vi "HMI.vi"() -> ()   [LabVIEW 2019, in "HMI Class 3.lvclass"]
uses:
  HMI Class 3.lvclass
  Control2.ctl
  Class 2.lvclass
  Datos Out.vi
  Datos In.vi
panel:
  out "mensajes a usuario":string
  in  "PARO DE E":bool
  in  "HISTORIAL DE FALLAS":bool
  in  "MODO AUTOMATICO":T1
  in  "Test":bool
  out "Numeric":dbl
  in  "MODO MANUAL":bool
  in  "stop":bool
  in  "INICIO":bool
  out "FALLA PRESENTE":bool
  out "MAQUINA EN ORIGEN":bool
  in  "RESET":bool
  in  "Tab Control":enum32{"0", "1", "2", "3", "4", "6", "7"}(tab)
  in  "MOVER A ORIGEN":bool
  out "PIEZA 2":bool
  out "PIEZA":bool
  in  "LIMITE MINIMO 2":dbl min=0.0 max=9999.0
  in  "LIMITE MAXIMO 2":dbl min=0.0 max=9999.0
  in  "LIMITE MINIMO":dbl min=0.0 max=9999.0
  in  "LIMITE MAXIMO":dbl min=0.0 max=9999.0
  out "ESTADO DE PIEZA TENSION":string
  out "ESTADO DE PIEZA GAP":string
  out "VALOR DE DISTANCIA":dbl
  in  "EST 2":bool
  out "SIN CAMBIOS":bool
  out "CON CAMBIOS":bool
  in  "EST 3":bool
  out "VALOR DE TENSIÓN":dbl
  in  "EST 1":bool
  out "SMAC SEGURO":bool
  out "PIEZA EN NIDO":bool
  in  "MANUAL":bool
  out "SMAC MUESTRA":bool
  out "SMAC APROX":bool
  in  "SMAC AVANZANDO":bool
  in  "SMAC RETORNANDO":bool
  in  "CILINDRO 2":bool
  in  "CILINDRO 1":bool
  out "SMAC AV. SEGURO":bool
  out "SMAC HOME":bool
  out "BIMANUAL 2":bool
  out "BIMANUAL 1":bool
  out "AVANCE CILINDRO 2":bool
  out "HOME CILINDRO 2":bool
  out "AVANCE CILINDRO 1":bool
  out "HOME CILINDRO 1":bool
  in  "ESTADISTICAS DE PRODUCCION":bool
  in  "CONFIGRUARCION DE PARAMETROS":bool
  in  "MODO DE OPERACION 2":bool
  # "MENÚ PRINCIPAL"
  # "MODO DE OPERACIÓN"
  # "ESTACION 1\n PRUEBA TENSIÓN"
  # "ESTACION 2\n PRUEBA GAP"
  # "ESTACION 3\n PRUEBA TRIP-GAP"
  # "CONTINUAIDAD EN CONTACTOS"
  # "PRODUCCIÓN"
  # "SENSORES"
  # "CILINDROS"
  # "SEGURIDAD"
  # "ESTADO DEL SMAC"
  # "SMAC"
  # "ENTRADAS                        SALIDAS"
  # "CONFIGURACION DE PARAMETROS"
  # "ESTADISTICAS DE PRODUCCIÓN"
  # "HISTORIAL DE FALLAS"
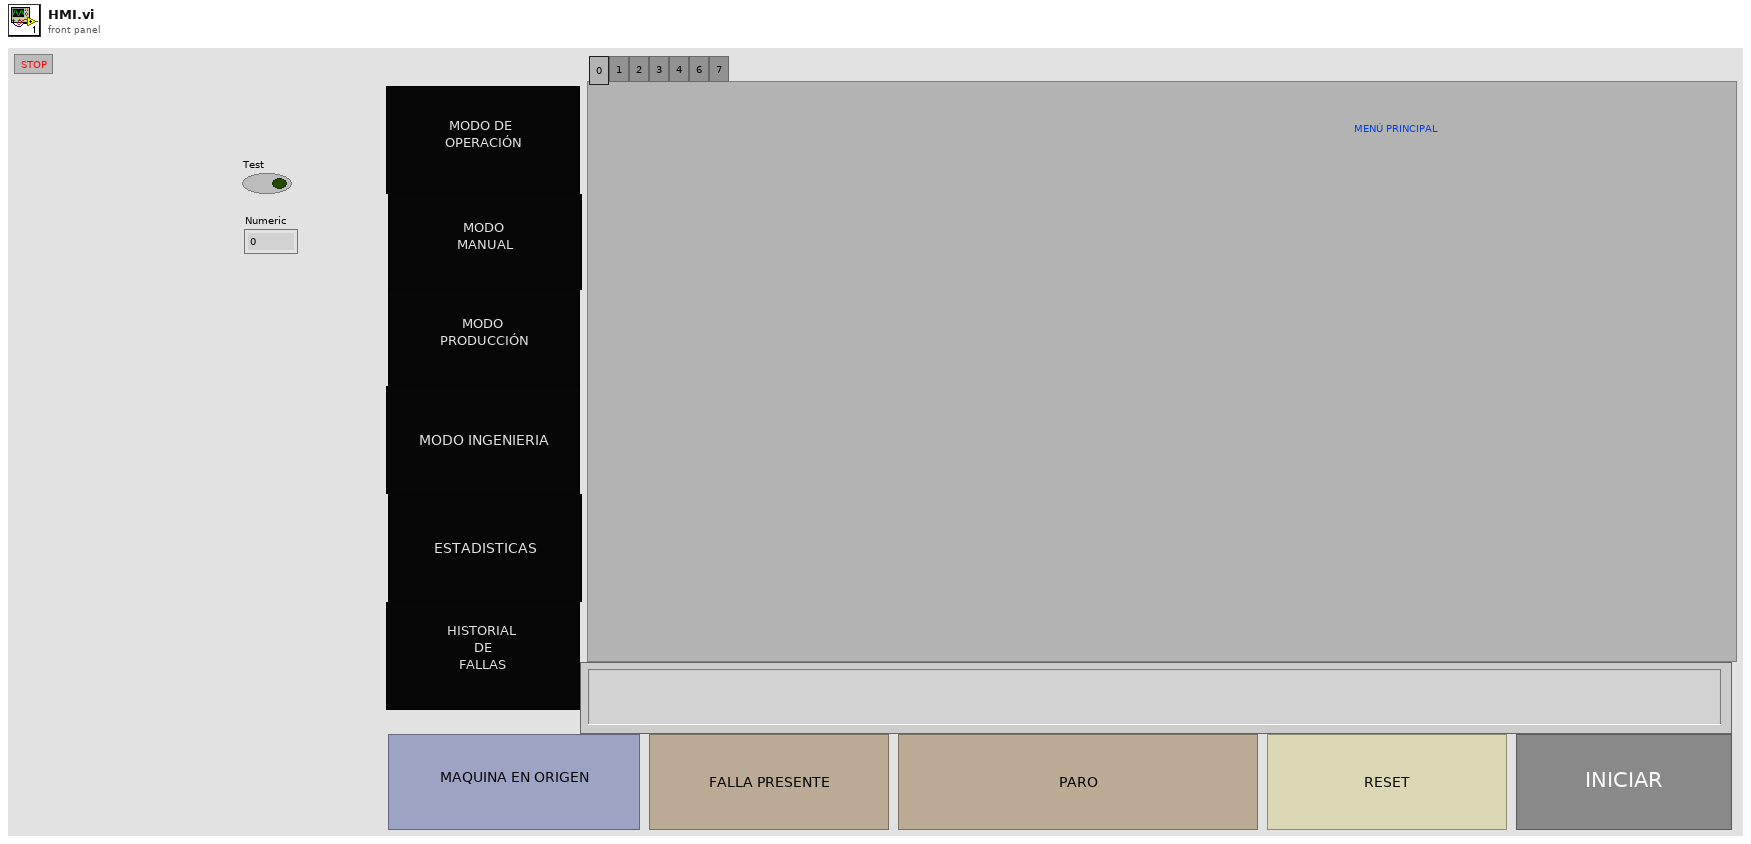
[diagram p1: front panel]
types:
  T1 = typedef "Control2.ctl" = bool
  T2 = cluster{"Test":bool, "CILINDRO _1":bool, "CILINDRO _2":bool, "SMAC_RETORNANDO":bool, "SMAC_AVANZANDO":bool, "MANUAL":bool, "EST_1":bool, "EST_2":bool, "EST_3":bool, "MOVER A ORIGEN":bool, "RESET":bool, "PARO":bool, "INICIO":bool, "DATA_CONTROL":cluster{"ESTACION_1":cluster{"ACEPTADA":bool, "MAXIMO":dbl, "MINIMO":dbl, "LECTURA":dbl}, "ESTACION_2":cluster{"ACEPTADA":bool, "MAXIMO":dbl, "MINIMO":dbl, "LECTURA":dbl}, "ESTACION_3":cluster{"ACEPTADA":bool, "MAXIMO":dbl, "MINIMO":dbl, "LECTURA":dbl}}}
  T3 = cluster{"SALIDAS.CILINDRO 1":bool, "SALIDAS.CILINDRO 2":bool, "SALIDAS.SEMAC RETORNANDO":bool, "SALIDAS.SAMAC AVANZANDO":bool, "Auto(off)/Manual(on)":bool, "HOME_CILINDRO_1":bool, "HOME_CILINDRO_2":bool, "AVANCE_CILINDRO_1":bool, "AVANCE_CILINDRO_2":bool, "PIEZA_EN_NIDO":bool, "BIMANUAL 2":bool, "BIMANUAL1":bool, "SIN CAMBIOS":bool, "CON  CAMBIOS":bool, "TESTER":bool, "MAQUINA EN ORIGEN":bool, "FALLA PRESENTE":bool}
  T4 = cluster{"Numeric":dbl, "VALOR DE DISTANCIA":dbl, "VALOR DE TENSION":dbl}
  T5 = cluster{"DATO GAP":string, "DATO TENSION":string, "mensajes usuario":string}
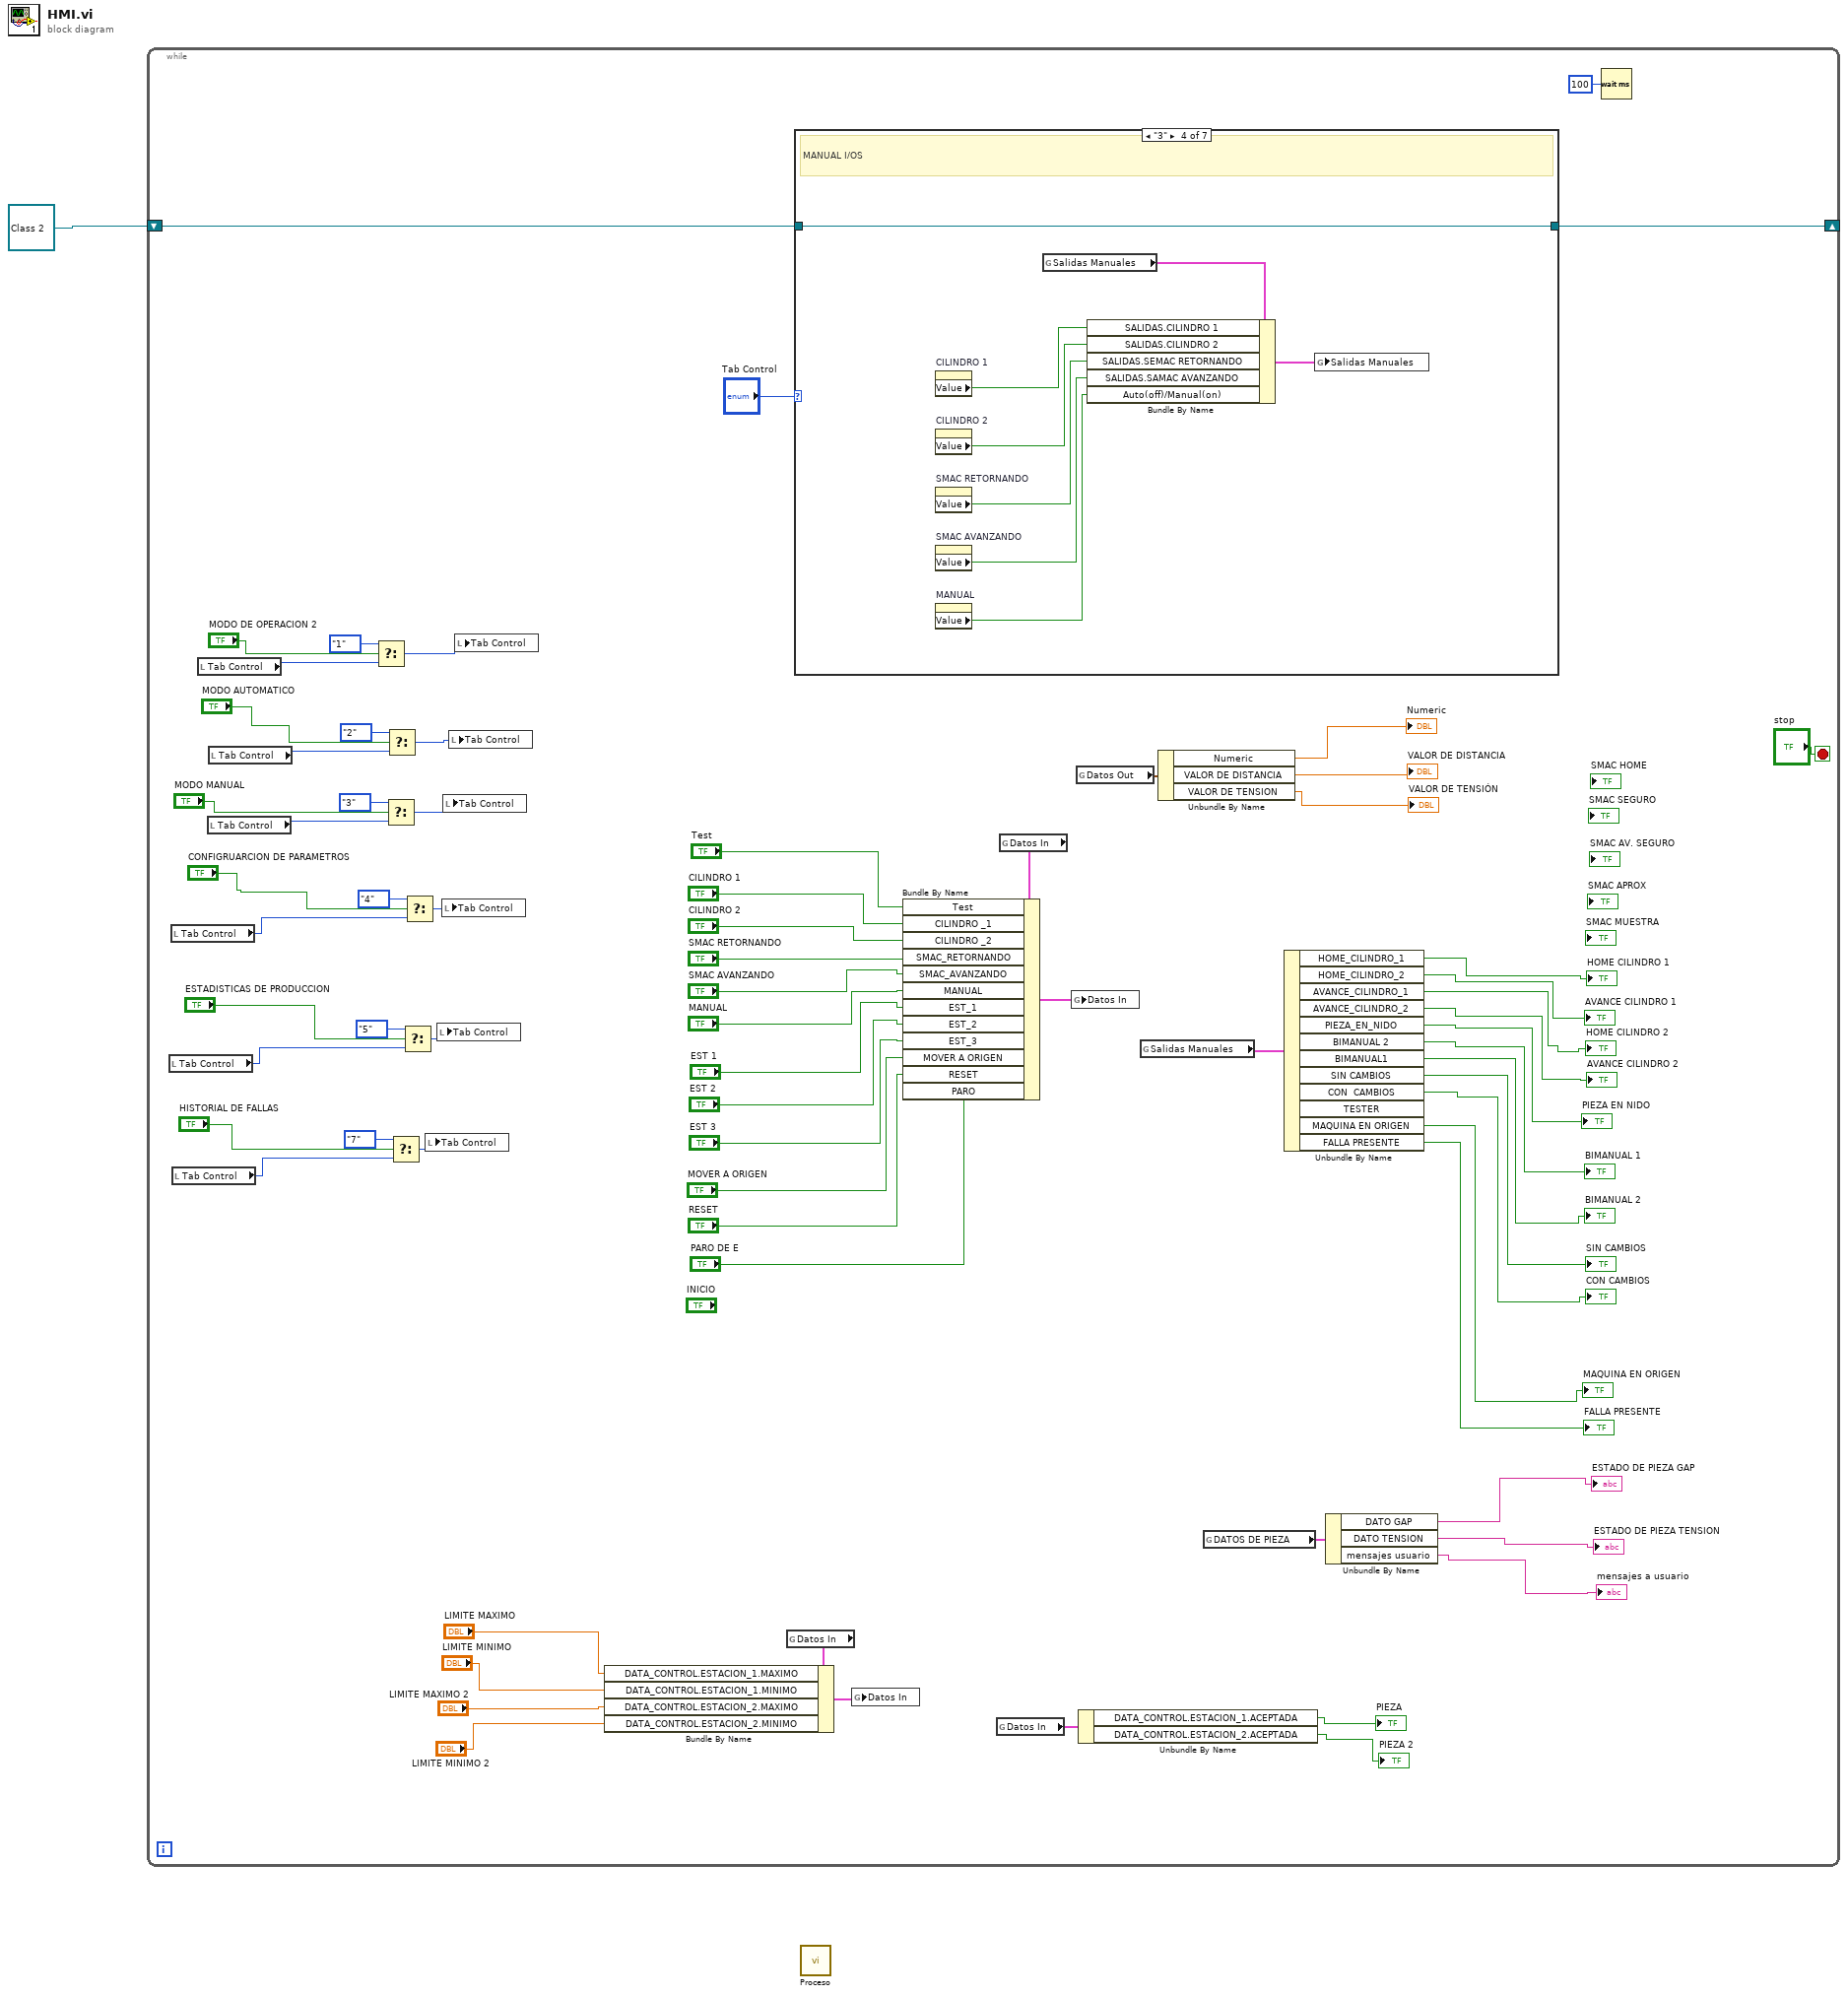
[diagram p0: block diagram]
diagram:
  n1 = while {
    shift-right: [w70] -> _
    shift-left: refnum<class "Class 2.lvclass"> refnum ("Class 2.lvclass") -> [w71]
    stop <- "stop" stop-if-true
    n2 = local read "Tab Control"() -> (w57:enum32{"0", "1", "2", "3", "4", "6", "7"})
    n3 = local read "Tab Control"() -> (w59:enum32{"0", "1", "2", "3", "4", "6", "7"})
    n4 = local read "Tab Control"() -> (w44:enum32{"0", "1", "2", "3", "4", "6", "7"})
    n5 = local read "Tab Control"() -> (w65:enum32{"0", "1", "2", "3", "4", "6", "7"})
    n6 = local read "Tab Control"() -> (w63:enum32{"0", "1", "2", "3", "4", "6", "7"})
    n7 = local read "Tab Control"() -> (w61:enum32{"0", "1", "2", "3", "4", "6", "7"})
    n8 = Select(t=enum32{"0", "1", "2", "3", "4", "5", "6", "7"}."1", s="MODO DE OPERACION 2", f=w65) -> (s? t:f=w51:u32)
    n9 = Select(t=enum32{"0", "1", "2", "3", "4", "5", "6", "7"}."3", s="MODO MANUAL", f=w63) -> (s? t:f=w47:u32)
    n10 = Select(t=enum32{"0", "1", "2", "3", "4", "5", "6", "7"}."2", s="MODO AUTOMATICO", f=w61) -> (s? t:f=w48:u32)
    n11 = Select(t=enum32{"0", "1", "2", "3", "4", "5", "6", "7"}."7", s="HISTORIAL DE FALLAS", f=w44) -> (s? t:f=w46:u32)
    n12 = Select(t=enum32{"0", "1", "2", "3", "4", "5", "6", "7"}."5", s="ESTADISTICAS DE PRODUCCION", f=w57) -> (s? t:f=w50:u32)
    n13 = Select(t=enum32{"0", "1", "2", "3", "4", "5", "6", "7"}."4", s="CONFIGRUARCION DE PARAMETROS", f=w59) -> (s? t:f=w49:u32)
    n14 = local write "Tab Control"(w46) -> ()
    n15 = local write "Tab Control"(w50) -> ()
    n16 = local write "Tab Control"(w49) -> ()
    n17 = local write "Tab Control"(w47) -> ()
    n18 = local write "Tab Control"(w48) -> ()
    n19 = local write "Tab Control"(w51) -> ()
    n20 = global read "Datos In.vi" "Datos In"() -> (w10:T2)
    n21 = Bundle By Name(cluster=w10, "DATA_CONTROL.ESTACION_1.MAXIMO"="LIMITE MAXIMO", "DATA_CONTROL.ESTACION_1.MINIMO"="LIMITE MINIMO", "DATA_CONTROL.ESTACION_2.MAXIMO"="LIMITE MAXIMO 2", "DATA_CONTROL.ESTACION_2.MINIMO"="LIMITE MINIMO 2") -> (w9:T2)
    n22 = case shown="\"3\"" "Tab Control" {
      tunnel: w71 -> [w74 w75 w76 w84 w85 w86 w87]
      tunnel: [w74 w75 w76 w84 w85 w86 w87] -> w70
      frame "0", Default {
        # "MENU PRINCIPAL"
      }
      frame "1" {
        # "MODO OPERACION"
      }
      frame "2" {
        # "MODO PRODUCCION"
      }
      frame "3" {
        # "MANUAL I/OS"
        n23 = property on="CILINDRO 1" class="Bool (strict)"() -> ("Value"=w83:bool)  [unwired: 2 in, 2 out]
        n24 = property on="CILINDRO 2" class="Bool (strict)"() -> ("Value"=w82:bool)  [unwired: 2 in, 2 out]
        n25 = property on="SMAC RETORNANDO" class="Bool (strict)"() -> ("Value"=w81:bool)  [unwired: 2 in, 2 out]
        n26 = property on="SMAC AVANZANDO" class="Bool (strict)"() -> ("Value"=w80:bool)  [unwired: 2 in, 2 out]
        n27 = property on="MANUAL" class="Bool (strict)"() -> ("Value"=w79:bool)  [unwired: 2 in, 2 out]
        n28 = global read "Datos Out.vi" "Salidas Manuales"() -> (w78:T3)
        n29 = Bundle By Name(cluster=w78, "SALIDAS.CILINDRO 1"=w83, "SALIDAS.CILINDRO 2"=w82, "SALIDAS.SEMAC RETORNANDO"=w81, "SALIDAS.SAMAC AVANZANDO"=w80, "Auto(off)/Manual(on)"=w79) -> (w77:T3)
        n30 = global write "Datos Out.vi" "Salidas Manuales"(w77) -> ()
      }
      frame "4" {
        # "CONFIGURACION DE PARAMETROS"
      }
      frame "6" {
        # "ESTADISTICAS DE PRODUCCION"
      }
      frame "7" {
        # "HISTORIAL DE FALLAS"
      }
    }
    n31 = global write "Datos In.vi" "Datos In"(w9) -> ()
    n32 = global read "Datos In.vi" "Datos In"() -> (w4:T2)
    n33 = global read "Datos In.vi" "Datos In"() -> (w17:T2)
    n34 = Bundle By Name(cluster=w17, "Test"="Test", "CILINDRO _1"="CILINDRO 1", "CILINDRO _2"="CILINDRO 2", "SMAC_RETORNANDO"="SMAC RETORNANDO", "SMAC_AVANZANDO"="SMAC AVANZANDO", "MANUAL"="MANUAL", "EST_1"="EST 1", "EST_2"="EST 2", "EST_3"="EST 3", "MOVER A ORIGEN"="MOVER A ORIGEN", "RESET"="RESET", "PARO"="PARO DE E") -> (w16:T2)
    n35 = global write "Datos In.vi" "Datos In"(w16) -> ()
    n36 = global read "Datos Out.vi" "Datos Out"() -> (w68:T4)
    n37 = Unbundle By Name(w4) -> ("DATA_CONTROL.ESTACION_1.ACEPTADA"=→"PIEZA":bool, "DATA_CONTROL.ESTACION_2.ACEPTADA"=→"PIEZA 2":bool)
    n38 = global read "Datos Out.vi" "Salidas Manuales"() -> (w31:T3)
    n39 = Unbundle By Name(w68) -> ("Numeric"=→"Numeric":dbl, "VALOR DE DISTANCIA"=→"VALOR DE DISTANCIA":dbl, "VALOR DE TENSION"=→"VALOR DE TENSIÓN":dbl)
    n40 = global read "Datos Out.vi" "DATOS DE PIEZA"() -> (w14:T5)
    n41 = Unbundle By Name(w31) -> ("HOME_CILINDRO_1"=→"HOME CILINDRO 1":bool, "HOME_CILINDRO_2"=→"AVANCE CILINDRO 1":bool, "AVANCE_CILINDRO_1"=→"HOME CILINDRO 2":bool, "AVANCE_CILINDRO_2"=→"AVANCE CILINDRO 2":bool, "PIEZA_EN_NIDO"=→"PIEZA EN NIDO":bool, "BIMANUAL 2"=→"BIMANUAL 1":bool, "BIMANUAL1"=→"BIMANUAL 2":bool, "SIN CAMBIOS"=→"SIN CAMBIOS":bool, "CON  CAMBIOS"=→"CON CAMBIOS":bool, "MAQUINA EN ORIGEN"=→"MAQUINA EN ORIGEN":bool, "FALLA PRESENTE"=→"FALLA PRESENTE":bool)  [unwired: 1 out]
    n42 = Unbundle By Name(w14) -> ("DATO GAP"=→"ESTADO DE PIEZA GAP":string, "DATO TENSION"=→"ESTADO DE PIEZA TENSION":string, "mensajes usuario"=→"mensajes a usuario":string)
    n43 = Wait (ms)(milliseconds to wait=u32 100) -> ()  [unwired: 1 out]
  }
  n44 = call "Proceso.vi"() -> ()  [unwired: 12 in]
